vi "SMU_Output Control.vi"(0 "Semiconductor Module Context":T1, 2 "output enabled?":bool, 5 "Pins":string[](array[string]), 11 "error in (no error)":errorcluster) -> (4 "Semiconductor Module Context Out":T1, 15 "error out":errorcluster)   [LabVIEW 2013]
uses:
  <vilib>/NI_TestStand_SemiconductorModule/NI_TestStand_Semiconductor_Module.lvlibp/PinMap/General/SemiconductorModuleContext.ctl
  <vilib>/NI_TestStand_SemiconductorModule/NI_TestStand_Semiconductor_Module.lvlibp/PinMap/DC Power/PinsToNIDCPowerSessions.vi
  <vilib>/NI_TestStand_SemiconductorModule/NI_TestStand_Semiconductor_Module.lvlibp
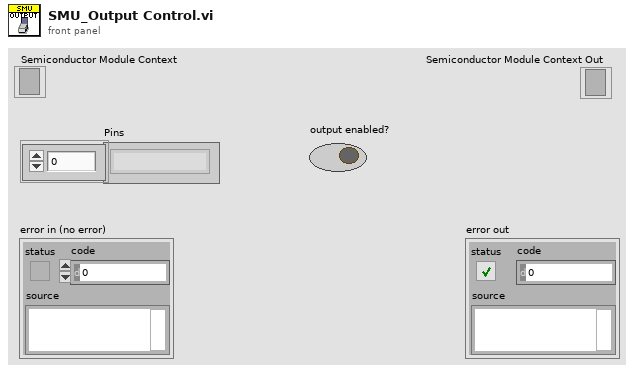
[diagram p1: front panel]
types:
  T1 = typedef "NI_TestStand_Semiconductor_Module.lvlibp/SemiconductorModuleContext.ctl" = refnum<k7>
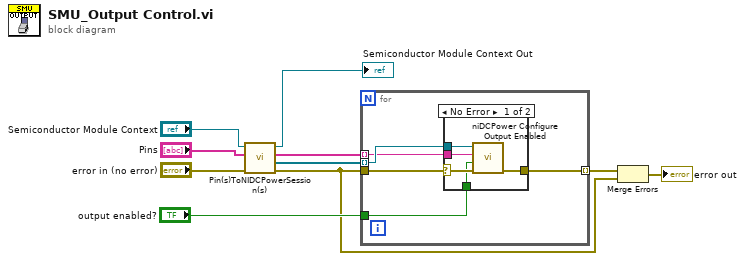
[diagram p0: block diagram]
diagram:
  n1 = call-poly <vilib>:"Pin(s)ToNIDCPowerSession(s).vi"("error in (no error)"="error in (no error)", "Pins"="Pins", "Semiconductor Module Context"="Semiconductor Module Context") -> ("error out"=w2:errorcluster, "Instrument Sessions"=w6:refnum<k15>[], "Channel Lists"=w7:string[], "Semiconductor Module Context Out"=→"Semiconductor Module Context Out":T1)  [unwired: 4 in, 1 out]
  n2 = for {
    tunnel: w2 -> [w15]
    tunnel: w7 -> [w13] mode=indexing
    tunnel: w6 -> [w14] mode=indexing
    tunnel: "output enabled?" -> [w12]
    tunnel: [w11] -> w3 mode=indexing
    n3 = case shown="No Error" w15 {
      selector: w15 -> [w20 w21]
      tunnel: [w19 w21] -> w11
      tunnel: w14 -> [w18 _]
      tunnel: w13 -> [w17 _]
      tunnel: w12 -> [w16 _]
      frame No Error {
        n4 = call <instrlib>:"niDCPower Configure Output Enabled.vi"("error in (no error)"=w20, "output enabled"=w16, "channel name"=w17, "instrument handle"=w18) -> ("error out"=w19:errorcluster)  [unwired: 6 in, 1 out]
      }
      frame Error {
      }
    }
  }
  n5 = Merge Errors(w3, w2) -> (→"error out":errorcluster)
